vi "layer.vi"(1 "weight":dbl[][](array[numeric])=[[0.1, 0.8, 0.4, 0.3], [0.2, 0.7, 0.4, 0.2], [0.3, 0.2, 0.1, 0.2]], 2 "Input":dbl[](array[numeric])=[1.0, 2.0, 3.0]) -> (0 "Output":dbl[](array[numeric]))   [LabVIEW 2009]
uses:
  <vilib>/Analysis/Matrix/Numeric/Conversions/Matrix To Array - RM.vi
  <vilib>/Analysis/Matrix/Numeric/Multiply/Multiply - RM,RM.vi
  <vilib>/Analysis/Matrix/Numeric/Conversions/Array To Matrix - RA2.vi
  <vilib>/Analysis/Matrix/Numeric/Conversions/Array To Matrix - RA.vi
  <vilib>/Analysis/Matrix/NI_Matrix.lvlib
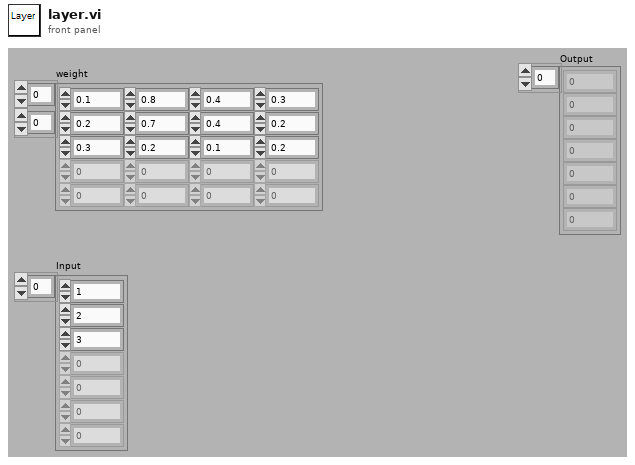
[diagram p1: front panel]
types:
  T1 = typedef "NI_Matrix.lvlib/RealMatrix.ctl" = dbl[][]
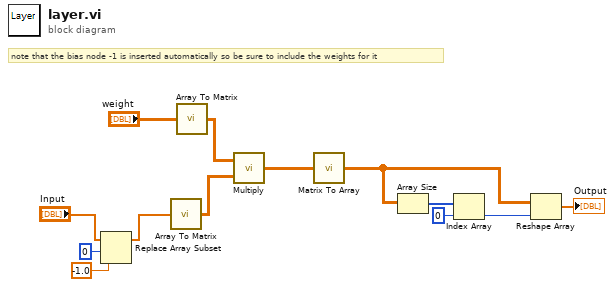
[diagram p0: block diagram]
diagram:
  # "note that the bias node -1 is inserted automatically so be sure to include the weights for it"
  n1 = Replace Array Subset(array="Input", new element=-1.0 ("new element/subarray"), index=0) -> (w1:dbl[])
  n2 = call-poly <vilib>:"Array To Matrix.vi"("Real 1D Array"=w1) -> ("Real Matrix (Column Vector)"=w12:T1)
  n3 = call-poly <vilib>:"Array To Matrix.vi"("Real 2D Array"="weight") -> ("Real Matrix"=w13:T1)
  n4 = call-poly <vilib>:"Multiply.vi"("Real Matrix B"=w12, "Real Matrix A"=w13) -> ("A * B"=w10:T1)
  n5 = call-poly <vilib>:"Matrix To Array.vi"("Real Matrix"=w10) -> ("Real 2D Array"=w8:dbl[][])
  n6 = Array Size(array=w8) -> (size(s)=w7:i32[])
  n7 = Index Array(array=w7, index=0) -> (element=w5:i32)
  n8 = Reshape Array(w8, w5) -> (→"Output":dbl[])
